vi "Set Test Node Project Path.vi"(8 "error in (no error)":errorcluster, 10 "Test Node Project Path":path, 11 "Test Node Model in":refnum<class "Test Node Model.lvclass">) -> (0 "error out":errorcluster, 3 "Test Node Model out":refnum<class "Test Node Model.lvclass">)   [LabVIEW 2013, in "Test Node Model.lvlib" / "Test Node Model.lvclass"]
uses:
  Test Node Model.lvclass
  Test Node Model.lvclass/Test Node Model.ctl
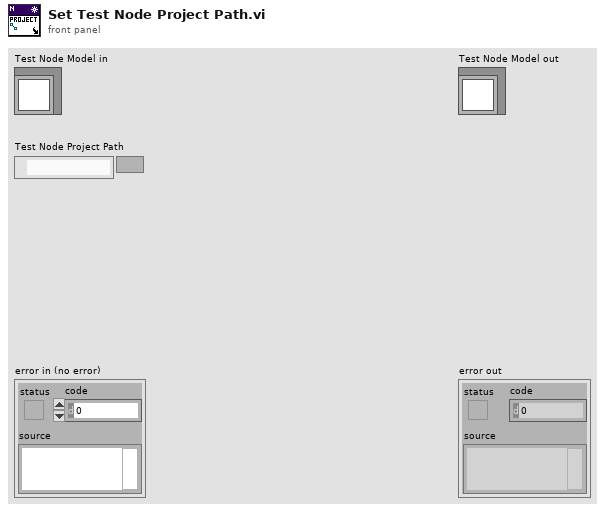
[diagram p1: front panel]
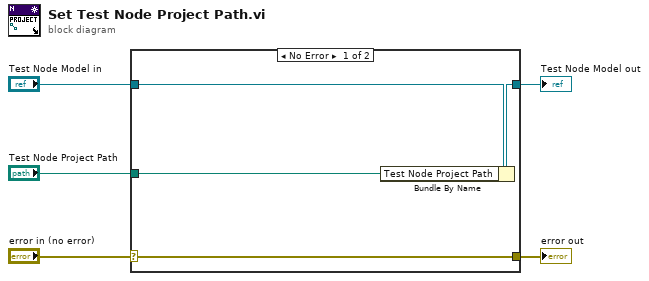
[diagram p0: block diagram]
diagram:
  n1 = case shown="No Error" "error in (no error)" {
    selector: "error in (no error)" -> [w9 w10]
    tunnel: [w9 w10] -> w4
    tunnel: [w7 w11] -> w2
    tunnel: "Test Node Model in" -> [w8 w11]
    tunnel: "Test Node Project Path" -> [w6 _]
    frame No Error {
      n2 = Bundle By Name(cluster=w8, "Test Node Project Path"=w6) -> (w7:refnum<class "Test Node Model.lvclass">)
    }
    frame Error {
    }
  }
  "error out" <- w4
  "Test Node Model out" <- w2
